vi "Config - Read.vi"(8 "error in (no error)":errorcluster, 11 "Config Data Array":T1[](array[typedef])) -> (0 "error out":errorcluster, 3 "Config Data Array":T1[](array[typedef]))   [LabVIEW 2017]
doc: "Reads the configuration data records"
uses:
  Controls/Config Data.ctl
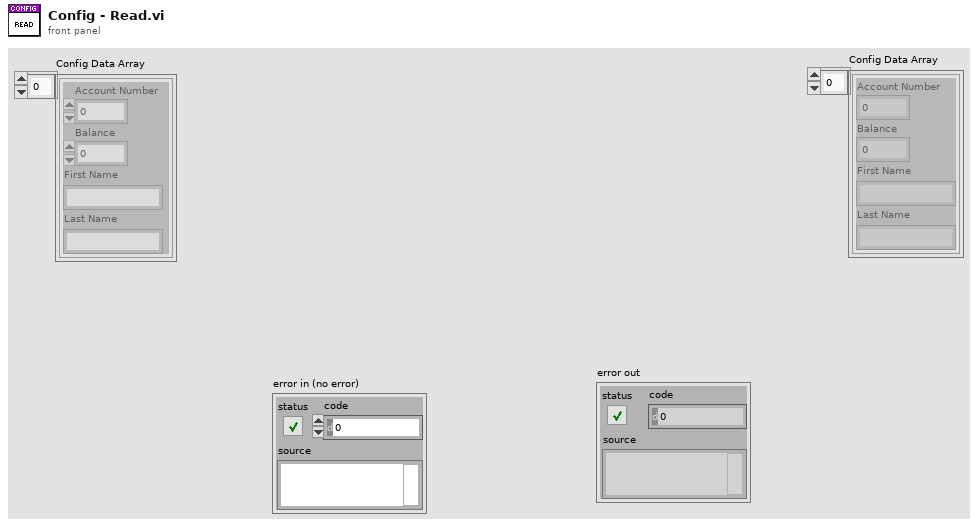
[diagram p1: front panel]
types:
  T1 = typedef "Config Data.ctl" = cluster{"Account Number":i32, "Balance":dbl, "First Name":string, "Last Name":string}
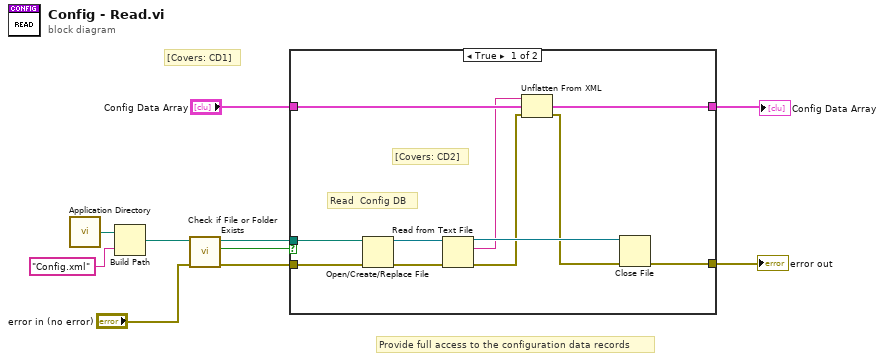
[diagram p0: block diagram]
diagram:
  # "[Covers: CD1]"
  # "Provide full access to the configuration data records"
  n1 = call <vilib>:"Application Directory.vi"() -> ("Application Directory"=w1:path)
  n2 = Build Path(base path=w1, name or relative path="Config.xml") -> (appended path=w10:path)
  n3 = call <vilib>:"Check if File or Folder Exists.vi"("error in (no error)"="error in (no error)", "path"=w10) -> ("error out"=w6:errorcluster, "file or folder exists?"=w8:bool, "dup path"=w7:path)  [unwired: 7 in]
  n4 = case shown="True" w8 {
    tunnel: w7 -> [w15 _]
    tunnel: w6 -> [w16 w22]
    tunnel: "Config Data Array" -> [w14 w23]
    tunnel: [w12 w22] -> w5
    tunnel: [w11 w23] -> w3
    frame True {
      # "Read  Config DB"
      # "[Covers: CD2]"
      n5 = Open/Create/Replace File(file path (use dialog)=w15, error in=w16) -> (refnum out=w18:refnum<file>, error out=w17:errorcluster)  [unwired: 4 in, 1 out]
      n6 = Read from Text File(file (use dialog)=w18, error in=w17) -> (refnum out=w21:refnum<file>, text=w13:string, error out=w19:errorcluster)  [unwired: 2 in, 1 out]
      n7 = Unflatten From XML(xml string=w13, type=w14, error in (no error)=w19) -> (value=w11:T1[], error out=w20:errorcluster)
      n8 = Close File(refnum=w21, error in=w20) -> (error out=w12:errorcluster)  [unwired: 1 out]
    }
    frame False {
      # "[Covers: CD4]"
    }
  }
  "Config Data Array" <- w3
  "error out" <- w5
